vi "Process_Laser_Cabinet_Status.vi"(1 "Data":string) -> (0 "output cluster 2":T1)   [LabVIEW 2023]
uses:
  TypeDefs/laser_cabinet_status.ctl
  <vilib>/Utility/Data Type/NI_Data Type.lvlib
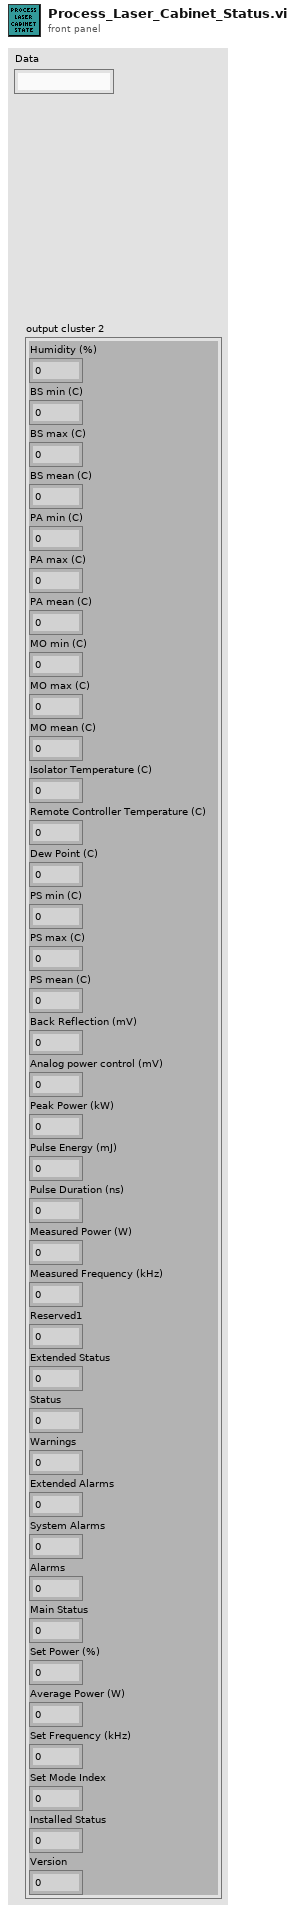
[diagram p1: front panel]
types:
  T1 = typedef "laser_cabinet_status.ctl" = cluster{"Version":u16, "Installed Status":u32, "Set Mode Index":u16, "Set Frequency (kHz)":sgl, "Average Power (W)":sgl, "Set Power (%)":sgl, "Main Status":u32, "Alarms":u32, "System Alarms":u32, "Extended Alarms":u32, "Warnings":u32, "Status":u32, "Extended Status":u32, "Reserved1":u16, "Measured Frequency (kHz)":sgl, "Pulse Duration (ns)":u32, "Measured Power (W)":sgl, "Pulse Energy (mJ)":sgl, "Peak Power (kW)":sgl, "Analog power control (mV)":sgl, "Back Reflection (mV)":sgl, "PS mean (C)":sgl, "PS max (C)":sgl, "PS min (C)":sgl, "Dew Point (C)":sgl, "Remote Controller Temperature (C)":sgl, "Isolator Temperature (C)":sgl, "MO mean (C)":sgl, "MO max (C)":sgl, "MO min (C)":sgl, "PA mean (C)":sgl, "PA max (C)":sgl, "PA min (C)":sgl, "BS mean (C)":sgl, "BS max (C)":sgl, "BS min (C)":sgl, "Humidity (%)":sgl}
  T2 = typedef "NI_Data Type.lvlib/Data Type.ctl" = enum8{"Invalid Type", "Void", "I8", "I16", "I32", "I64", "U8", "U16", "U32", "U64", "Single Float", "Double Float", "Extended Float", "Single Complex", "Double Complex", "Extended Complex", "Enum U8", "Enum U16", "Enum U32", "Enum U64", "Single Float With Unit", "Double Float With Unit", "Extended Float With Unit", "Single Complex with Unit", "Double Complex with Unit", "Extended Complex with Unit", "Boolean", "String", "Path", "Picture", "Tag", "Array", "Cluster", "Variant", "LV Variant", "Waveform", "Timestamp", "Digital Waveform", "Digital Data", "ExpressData", "Refnum", "External Data", "VI", "Poly VI", "LabVIEW Class Instance", "Fixed Point", "Set Collection", "Map Collection"}
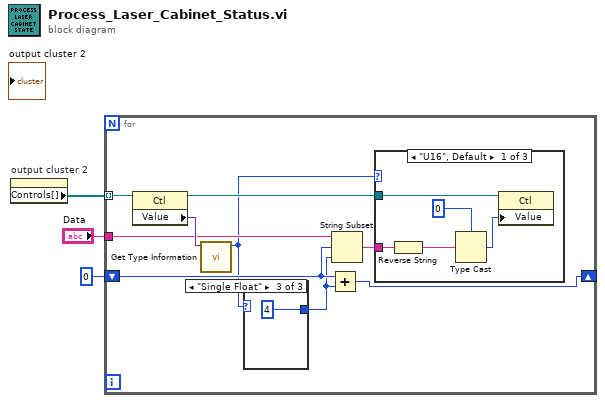
[diagram p0: block diagram]
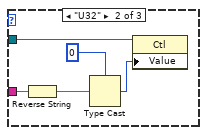
[diagram p2: hidden frame]
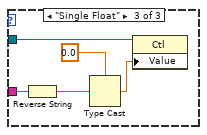
[diagram p3: hidden frame]
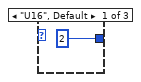
[diagram p4: hidden frame]
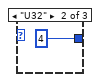
[diagram p5: hidden frame]
diagram:
  n1 = property on="output cluster 2" class="Clust (strict)"() -> ("Controls[]"=w3:refnum<vi>[])  [unwired: 2 in, 2 out]
  n2 = for {
    tunnel: w3 -> [w12] mode=indexing
    tunnel: "Data" -> [w10]
    shift-right: [w7] -> _
    shift-left: 0 -> [w9]
    n3 = property class="Ctl"(reference=w12) -> (reference out=w5:refnum<vi>, "Value"=w11:variant)  [unwired: 1 in, 1 out]
    n4 = call <vilib>:"Get Type Information.vi"("variant"=w11) -> ("type"=w4:T2)  [unwired: 6 in, 4 out]
    n5 = case shown="\"Single Float\"" w4 {
      tunnel: [2 4 4] -> w8
      frame "U16", Default {
      }
      frame "U32" {
      }
      frame "Single Float" {
      }
    }
    n6 = Add(x=w9, y=w8) -> (x+y=w7:i32)
    n7 = String Subset(string=w10, offset (0)=w9, length (rest)=w8) -> (substring=w6:string)
    n8 = case shown="\"U16\", Default" w4 {
      tunnel: w6 -> [w16 w20 w25]
      tunnel: w5 -> [w13 w19 w24]
      frame "U16", Default {
        n9 = Reverse String(1:w16) -> (0:w17:string)
        n10 = Type Cast(type=u16 0, x=w17) -> (*(type *) &x=w14:u16)
        n11 = property class="Ctl"(reference=w13, "Value"=w14) -> ()  [unwired: 1 in, 2 out]
      }
      frame "U32" {
        n12 = Reverse String(1:w20) -> (0:w22:string)
        n13 = Type Cast(type=u32 0, x=w22) -> (*(type *) &x=w18:u32)
        n14 = property class="Ctl"(reference=w19, "Value"=w18) -> ()  [unwired: 1 in, 2 out]
      }
      frame "Single Float" {
        n15 = Reverse String(1:w25) -> (0:w27:string)
        n16 = Type Cast(type=sgl 0.0, x=w27) -> (*(type *) &x=w23:sgl)
        n17 = property class="Ctl"(reference=w24, "Value"=w23) -> ()  [unwired: 1 in, 2 out]
      }
    }
  }
